vi "Keseluruhan Sistem.vi"() -> ()   [LabVIEW 2011]
doc: "The Basic Serial Read and Write example performs a Serial Port Read, a Serial Port Write, or a combination of these actions. The user selects the actions (read or write) on the front panel. If both are selected, the VI will write the data first, read data, and then close the VISA session that is opened to the port. This VI will wait until the specified number of bytes is received at the port. Only the number of bytes specified will be read.\n\nINSTRUCTIONS:\n1) Select the serial resource and configuration parameters (baud rate, data bits, parity, stop bits, flow control).\n2) Select the operations to be performed. \n3) Connect the serial port to your device. If no device is available, perform a loopback test by doing one of the following. Short pins 2 and 3 on a RS-232 cable or short pin 4 to pin 8 and pin 5 to pin 9 on a RS-485/422 cable. \n4) Run the VI to see the data read. (The \"read string\" will match the \"string to write\" if a loopback test was performed.)\n\nNote: The parameters set for the serial port must match the parameters of the connected instrument or device. In this example, the bytes to read parameter specifies the number of bytes that the serial port reads. If there were more bytes at the port than the number specified in bytes to read, those bytes would not be read. Also, if you specify to read more bytes than the number of bytes actually read, you might receive a timeout error message.\n\nOn the block diagram, the Configure Serial Port VI sets the configuration parameters. The front panel displays the controls used to configure the basic parameters, such as baud rate, data bits, and parity. Constants configure the other parameters the user probably does not need set. After the VISA Configure Serial Port VI opens the VISA session and configures the port, the VI passes the VISA resource name to other VIs that perform operations on that VISA resource. The VISA Write function sends a command to the serial device and the VISA Read function returns data based on the command. The VISA Close function then closes the reference to the serial device. It is important to close the reference; otherwise communication through with that port through protocols other than VISA might not be possible."
uses:
  <vilib>/Simulation/Scripting/Companion Diagram/SimConfigNode/SimParams.ctl
  <vilib>/Simulation/Scripting/Companion Diagram/SimConfigNode/_simSolvers.ctl
  <vilib>/Simulation/Implementation/Shared/SIMSCR Execution Mode.ctl
  <vilib>/Simulation/Param Hierarchy/Typedefs/SIMPH Param Control Actions.ctl
  <vilib>/Simulation/Implementation/Shared/NILVSim_FinalizeModel.vi
  <vilib>/Simulation/Implementation/Shared/NILVSim_Manager.vi
  <vilib>/Simulation/Implementation/Shared/NILVSim_ParamChanged.vi
  <vilib>/imath/engines/lvmath2/RunTimeEngine/ErrorHandling/NIMS_Finalize Error.vi
  <vilib>/imath/engines/lvmath2/RunTimeEngine/BuiltInFunctions/deg_to_rad/NIMS_deg_to_rad.vi
  <instcachedir>/0/NIMS_deg_to_rad_4A81D684CE8D4DD79924F5AB74D756E1.lvgen/NIMS_deg_to_rad_4A81D684CE8D4DD79924F5AB74D756E1_001.vi
  <vilib>/imath/engines/lvmath2/RunTimeEngine/NodeEndStatement/NIMS_NodeEndStatement_Output.vi
  <instcachedir>/0/NIMS_NodeEndStatement_Output_53EC0D466D134D7ABD903AC30B43404B.lvgen/NIMS_NodeEndStatement_Output_53EC0D466D134D7ABD903AC30B43404B_001.vi
  <instcachedir>/0/NIMS_NodeEndStatement_Output_53EC0D466D134D7ABD903AC30B43404B.lvgen/NIMS_NodeEndStatement_Output_53EC0D466D134D7ABD903AC30B43404B_012.vi
  <instcachedir>/0/NIMS_NodeEndStatement_Output_53EC0D466D134D7ABD903AC30B43404B.lvgen/NIMS_NodeEndStatement_Output_53EC0D466D134D7ABD903AC30B43404B_010.vi
  <vilib>/imath/engines/lvmath2/RunTimeSupport/NIMS_Complex To Real.vi
  <instcachedir>/0/NIMS_Complex To Real_C6C689ECDA084B0290AC275552CC3682.lvgen/NIMS_Complex To Real_C6C689ECDA084B0290AC275552CC3682_001.vi
  <vilib>/imath/engines/lvmath2/RunTimeEngine/BuiltInFunctions/rad_to_deg/NIMS_rad_to_deg.vi
  <instcachedir>/0/NIMS_rad_to_deg_A39AFCDDC8C049FCADAAB7FC30B9F5AA.lvgen/NIMS_rad_to_deg_A39AFCDDC8C049FCADAAB7FC30B9F5AA_001.vi
  <vilib>/imathl/engines/lvmath/Functions/Error Handling/Create Error.vi
  <vilib>/imath/engines/lvmath2/RunTimeEngine/BuiltInFunctions/abs/NIMS_abs(signed).vi
  <instcachedir>/0/NIMS_abs(signed)_C4FCB8E6058B49B797C7C8D53CA5F6EC.lvgen/NIMS_abs(signed)_C4FCB8E6058B49B797C7C8D53CA5F6EC_002.vi
  <vilib>/imath/engines/lvmath2/RunTimeEngine/BuiltInFunctions/acos/NIMS_acos(C).vi
  <instcachedir>/0/NIMS_acos(C)_7CE2F6FACE8F41D2AB6320A13102A19C.lvgen/NIMS_acos(C)_7CE2F6FACE8F41D2AB6320A13102A19C_001.vi
  <vilib>/Instr/_visa.llb/VISA Configure Serial Port (Instr).vi
  <vilib>/imath/engines/lvmath2/RunTimeEngine/Managers/WorkSpace/UID Generator.vi
  <vilib>/imath/engines/lvmath2/RunTimeEngine/Managers/SymbolTable/Clear UID.vi
  <instcachedir>/0/NIMS_abs(signed)_C4FCB8E6058B49B797C7C8D53CA5F6EC.lvgen/NIMS_abs(signed)_C4FCB8E6058B49B797C7C8D53CA5F6EC_007.vi
  <instcachedir>/0/NIMS_Complex To Real_C6C689ECDA084B0290AC275552CC3682.lvgen/NIMS_Complex To Real_C6C689ECDA084B0290AC275552CC3682_003.vi
  <vilib>/imath/engines/lvmath2/RunTimeEngine/RunTimeType/NIMS_RunTimeType_From StrictType (excl LVString).vi
  <instcachedir>/0/NIMS_RunTimeType_From StrictType (excl LVString)_46AE8B54A11948F0BCCEB8091EE7AA4C.lvgen/NIMS_RunTimeType_From StrictType (excl LVString)_46AE8B54A11948F0BCCEB8091EE7AA4C_000.vi
  <vilib>/imath/engines/lvmath2/RunTimeEngine/LocalVariableDefStatement/MC_LocalVariableDefStatement_Display.vi
  <vilib>/Simulation/Implementation/Shared/SIM Unbundle Sim Info.vi
  <vilib>/Simulation/Implementation/Shared/NILVSim_GetModelError.vi
  <vilib>/Simulation/Implementation/Shared/SIM Bundle Sim Info.vi
  <vilib>/Simulation/Implementation/Shared/NILVSim_Initialize.vi
  <vilib>/Simulation/Implementation/XNodeFramework/SimXNode/SimX.xnode
  <vilib>/Simulation/Model Libraries/PID/SIM PID (Academic).vi
  <vilib>/Simulation/Model Libraries/PID/SIM PID.vi
  <vilib>/Simulation/Scripting/Companion Diagram/SimConfigNode/SimDog.xnode
  <vilib>/vision/NI_Vision_Development_Module.lvlib
  <vilib>/Simulation/Implementation/Shared/NI_SIM_Implementation.lvlib
  <vilib>/imath/engines/lvmath2/RunTimeEngine/Managers/SymbolTable/NIMS_WorkSpace.lvlib
panel:
  in  "Color Plane":i32(ring)=1 items=["Red", "Green", "Blue", "Hue", "Saturation", "Luminance", "Value", "Intensity"]
  out "bytes read":u32
  out "read string":string
  out "error vision 2":errorcluster
  in  "STOP":bool caption="Stop (F)"
  out "error vision":errorcluster
  in  "OFFSET":dbl
  out "error out":errorcluster
  in  "error in":errorcluster
  in  "Tab Control":T1(tab)
  in  "Tab Control 2":T2(tab)
  in  "Tab Control 3":enum32{"Pengolahan Citra", "Kinematika"}(tab)
  in  "Settings":T3={"Objects"=1, "Threshold"=128, "Reject Border"=FALSE, "Fill Holes"=FALSE, "Min Object Size"=FALSE, "Min Size"=100, "Max Object Size"=FALSE, "Max Size"=10000, "Show Search Area"=FALSE, "Show Center"=TRUE, "Show Bounding Box"=TRUE} {"Objects" items=["Bright Objects", "Dark Objects"]; "Threshold" min=1 max=999999999 step=1; "Max Size" min=1 max=999999999 step=1; "Min Size" min=1 max=999999999 step=1}
  in  "Alamat Berkas":path=path "E:/D4 - TUGAS AKHIR/Programs/Praktikum/polman.png"
  out "Citra \nHitam/Putih":T4(plugin-control)
  out "Citra Asli":T4(plugin-control)
  out "Hasil\nSegmentasi":T4(plugin-control)
  out "Hasil \nKlasifikasi":T4(plugin-control)
  in  "BERKAS / KAMERA":bool
  out "Number of Objects":i32
  in  "Range":cluster{"Lower value":sgl, "Upper value":sgl}={"Lower value"=128.0, "Upper value"=255.0} {"Upper value" format="%.2f"; "Lower value" format="%.2f"}
  out "Objects":T5(array[cluster]) {"Aspect Ratio" format="%.2f"; "Orientation" format="%.2f"; "Area" format="%.2f"; "Object Center"."Y" format="%.2f"; "Object Center"."X" format="%.2f"}
  in  "Replace Value":sgl=255.0 format="%.2f"
  in  "Dimensi Lengan Robot":cluster{"l1":sgl, "l2":sgl, "l3":sgl, "l4":sgl}={"l1"=75.0, "l2"=95.0, "l3"=95.0, "l4"=107.0} caption="Arm Dimensiions 2"
  out "SIDE VIEW ROBOT":cluster{"Y":dbl[], "Y":dbl[]}[](graph)
  out "TOP VIEW ROBOT":cluster{"Y":dbl[], "Y":dbl[]}[](graph)
  in  "Kinematik Maju / Balik":enum32{"Kinematika Maju", "Kinematika Balik"}(tab)
  out "Koordinat Akhir (KM)":cluster{"X":dbl, "Y":dbl, "Z":dbl}
  in  "BASE":dbl(knob) scale=-90.0..90.0
  in  "SHOULDER":dbl(knob)=30.0 scale=0.0..135.0
  in  "ELBOW":dbl(knob)=150.0 scale=90.0..270.0
  in  "WRIST":dbl(knob)=150.0 scale=90.0..270.0
  in  "ELBOW CONFIG":bool
  in  "Koordinat Z":dbl(slide)=75.0 scale=0.0..300.0
  in  "Koordinat Y":dbl(slide) scale=-135.0..135.0
  in  "Koordinat X":dbl(slide)=297.0 scale=0.0..300.0
  out "Sudut Persendian (KB)":cluster{"q1":dbl, "q2":dbl, "q3":dbl, "q4":dbl}
  in  "theta":dbl(knob) scale=0.0..90.0
  in  "INTEGRATE":bool
  in  "PWM\nGRIPPER":i32
  in  "SETPOINT\nGAYA":dbl=35.0
  in  "FREEZE":bool caption="Stop (F)"
  in  "INITIAL":bool caption="Stop (F)"
  out "SIDE VIEW":cluster{"Y":dbl[], "Y":dbl[]}[](graph)
  in  "Drawing Mode":u32(ring) items=["Frame", "Fill", "Highlight"]
  out "Image":T4(plugin-control)
  in  "Color":u32(colorbox)=16711680
  out "Waveform Chart":dynamicdata(graph)
  in  "Arm Dimensiions":cluster{"l1":sgl, "l2":sgl, "l3":sgl, "l4":sgl}={"l1"=75.0, "l2"=95.0, "l3"=95.0, "l4"=107.0} caption="Arm Dimensiions 2"
  out "PWM Values":T6
  out "Joint Angles":cluster{"q1":dbl, "q2":dbl, "q3":dbl, "q4":dbl}
  in  "START":bool
  in  "buffer":string
  out "TOP VIEW":cluster{"Y":dbl[], "Y":dbl[]}[](graph)
  out "Z ROBOT":sgl
  out "Y ROBOT":sgl
  out "X ROBOT":sgl
  out "Z CAMERA":sgl
  out "X CAMERA":sgl
  out "Y CAMERA":sgl
  in  "WAIT TIME":u32=750
  in  "VISA NAME":refnum<visa-resource-name>="COM24"
  out "SHADOW":sgl
  in  "INDICATOR":bool
  in  "FORCE \nCONTROL":bool
  in  "SETPOINT\nPOSISI":i32=1250
  out "OUTPUT":dbl
  in  "Kp":dbl=0.7
  in  "Ti":dbl=1.55
  in  "Td":dbl
  in  "ERROR":dbl
  out "INPUT":u8
  # "Rancang Bangun Sistem Kendali Pergerakan Berbasis Pengolahan Citra \ndan Kendali Gaya Pencekaman Pada Model Robot Berlengan\nNur Jamiludin R. , Dr. Noval Lilansa, Dipl. Ing., MT. , Afaf Fadhil Rifa'i, ST. MT.\nJurusan Teknik Mesin dan Manufaktur Konsentrasi Teknik Elektromekanik.\nPoliteknik Manufaktur Negeri Bandung\nJl. Kanayakan No. 21, Bandung 40135\nINDONESIA\nEmail : nur_jamiludin@elmecs-indonesia.com"
  # "Deskripsi\n\nSebuah robot berlengan mampu melakukan pekerjaan pemindahan obyek. Kebanyakan robot memiliki waktu operasi yang tidak efisien karena membutuhkan proses masukan koordinat tujuan oleh operator. Selain permasalahan tersebut masalah robot berlengan terbesar ialah bahwa saat robot melakukan tugas pemindahan obyek, robot tersebut berpotensi merusak obyek yang dipindahkan. Dibutuhkan sistem kendali pergerakan robot yang memiliki kemampuan pendeteksian obyek berbasis pengolahan citra, sehingga robot mampu menentukan koordinat tujuan secara otomatis. \n\nProgram ini merupakan program pengendali model robot berlengan lynxmotion L5AC yang terintegrasi pada sebuah kamera dengan resolusi 3.0 Megapixel dan perangkat keras SSC (Serial Servo Controller). Program kendali robot berlengan ini bertujuan mengendalikan sistem agar dapat mendeteksi obyek berbentuk bola secara otomatis, serta dapat memindahkan obyek tersebut tanpa menimbulkan cacat bentuk pada objek."
  # "Citra asli hasil \ntangkapan kamera"
  # "Berkaitan dengan persiapan pengolahan citra. \nIdentifikasi spesifikasi resolusi kamera\nPenentuan peletakkan titik pusat lensa kamera\nPenentuan ukuran hasil citra (image) yang diambil"
  # "Prepocessing"
  # "hasil segmentasi"
  # "Segmentasi menggunakan metode tresholding.\nProses tresholding mengubah citra dengan format gray-scale menjadi citra biner untuk memisahkan obyek pada citra dengan latar belakangnya."
  # "Segmentasi"
  # "Koordinat obyek hasil estimasi posisi merupakan koordinat dengan titik pusat area kerja sebagai referensi\nPindahkan referensinya menjadi titik pusat robot sebagai referensi"
  # "hasil klasifikasi"
  # "Ekstraksi ciri mencari obyek dengan karakteristik tertentu dari data citra yang diperoleh. \nKlasifikasi menentukan obyek dari informasi citra yang diolah dengan perhitungan matematis berdasarkan karakter fisik obyek."
  # "Ekstraksi Ciri\ndan Klasifikasi"
  # "Estimasi posisi  mendapatkan vektor posisi pusat massa obyek  terhadap pusat kerangka koordinat area kerja. \nKemudian dilakukan translasi pusat kerangka koordinat area kerja ke pusat kerangka koordinat base robot,"
  # "Estimasi Posisi"
  # "hasil estimasi posisi"
  # "Transformasi Homogen"
  # "tentukan kerangka koordinat tiap joint"
  # "konstruksi model robot"
  # "tentukan panjang link dan link offset"
  # "Parameter D-H\n(Denavit-Hattenberg)"
  # "tentukan link twist , joint angle merupakan variable"
  # "pemodelan stick diagram"
  # "Algoritma Perhitungan Matrix"
  # "Analisa Geometri"
  # "Pengendalian gaya yang digunakan pada sistem pada dasarnya merupakan pengendalian posisi bukaan gripper\nPosisi bukaan gripper merupakan fungsi dari gaya yang diakuisisi oleh sensor dikali dengan koefisien peredam (damper). pada sistem kendali dalam tugas akhir ini, koefisien peredam yang dimaksud merupakan karakteristik mekanik dari model lengan robot yang digunakan.\nPengendalian posisi dipilih mengingat penggerak gripper merupakan motor servo yang bergerak berdasarkan setpoint posisi."
  # "Percobaan kinematika maju ini didasarkan pada konfigurasi robot berlengan yang terintegrasi dengan sistem. \nRobot yang digunakan merupakan robot revolute yang memiliki 4 DOF ditambah satu gripper.\nRentang sudut yang diperbolehkan juga berdasarkan karakteristik penggerak robot\n\nParameter D-H  robot dapat dilihat pada tabel disamping."
  # "Percobaan kinematika balik ini merupakan perhitungan balik dari \npercobaan kinematika maju pada tab sebelumnya.\nsolusi kinematika balik yang beragam ditampilkan pada simulasi\ndengan memilih konfigurasi elbow up atau elbow down \nnamun robot berlengan yang terintegrasi dengan sistem hanya \nmenggunakan konfigurasi elbow up"
  # "mm"
  # "mm"
  # "mm"
  # "mm"
  # "mm"
  # "mm"
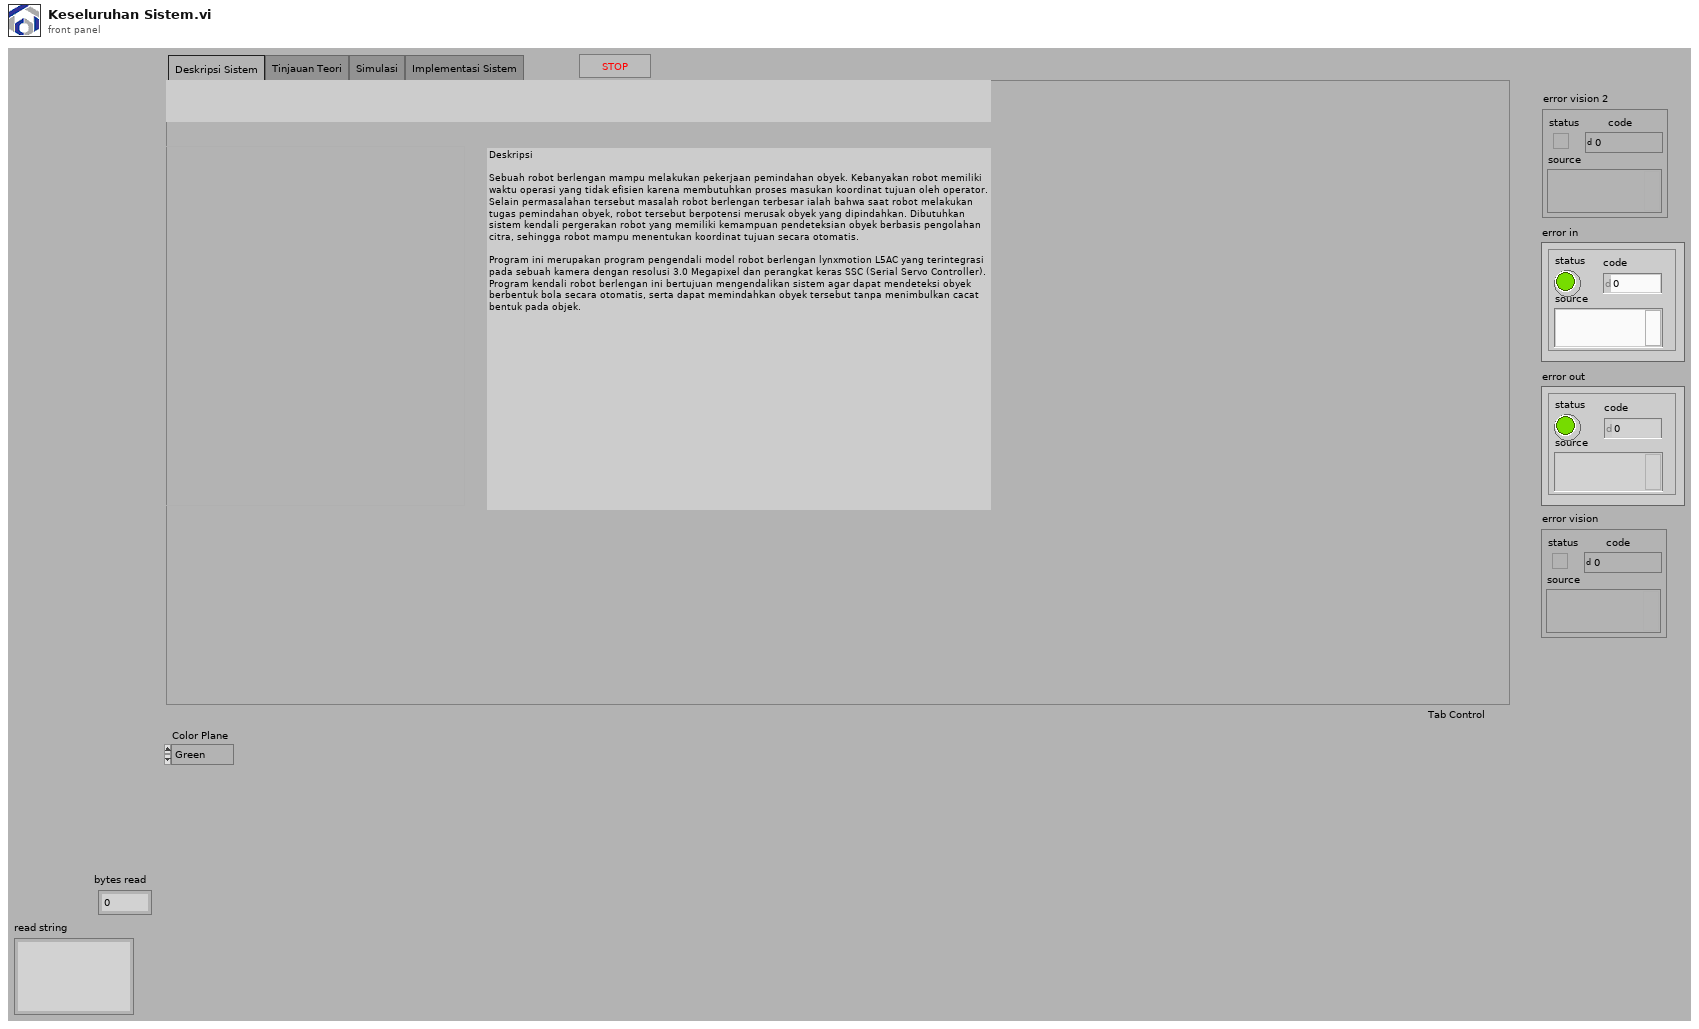
[diagram p1: front panel]
types:
  T1 = enum32{"Deskripsi Sistem", "Tinjauan Teori", "Simulasi", "Implementasi Sistem"}
  T2 = enum32{"Pengolahan Citra", "Kinematika Maju", "Kinematika Balik", "Pengendalian Gaya"}
  T3 = cluster{"Objects":u16, "Threshold":i32, "Reject Border":bool, "Fill Holes":bool, "Min Object Size":bool, "Min Size":i32, "Max Object Size":bool, "Max Size":i32, "Show Search Area":bool, "Show Center":bool, "Show Bounding Box":bool}
  T4 = typedef "IMAQ Image.ctl" = refnum<image>
  T5 = cluster{"Object Center":cluster{"X":sgl, "Y":sgl}, "Bounding Box":cluster{"X Left":i32, "Y Top":i32, "X Right":i32, "Y Bottom":i32}, "Area":sgl, "Orientation":sgl, "Aspect Ratio":sgl, "Nb Holes":i32}[]
  T6 = cluster{"PWM1":u32, "PWM2":u32, "PWM3":u32, "PWM4":u32}
  T7 = typedef "Image Type" = u32
  T8 = typedef "SIMPH Param Control Actions.ctl" = enum16{"get params", "set params"}
  T9 = typedef "SimParams.ctl" = cluster{"Initial Time (s)":dbl, "Final Time (s)":dbl, "Step Size (s)":dbl, "ODE Solver":T10, "Minimum Step Size (s)":dbl, "Maximum Step Size (s)":dbl, "Relative Tolerance":dbl, "Absolute Tolerance":dbl, "Software Timing":bool, "Initial Step Size (s)":dbl, "Automatic Fixed Step Size?":bool, "Automatic Discrete Step Size?":bool, "Discrete Step Size (s)":dbl, "Calculate using Time Step":bool, "Solver Wired?":bool, "Prev.Frm.Expected End":u64, "Prev.Frm.Actual End":u64, "Prev.Frm.Finished Late?":bool, "Prev.Iter.Expected End":u64, "Prev.Iter.Actual End":u64, "Prev.Iter.Finished Late?":bool, "Expected Iteration Start":u64, "Actual Iteration Start":u64, "Expected Frame Start":u64, "Actual Frame Start":u64, "Source Name":string, "Name":string, "Period":i64, "Deadline":i64, "Offset":i64, "Start":i64, "Priority":i32, "Timeout":i32, "Processor":i32, "Mode":enum32{"No Change", "Process missed periods, maintain original phase", "Discard missed periods, maintain original phase", "Process missed periods, ignore original phase", "Discard missed periods, ignore original phase"}, "Wakeup reason":enum32{"Normal", "Aborted", "Asynchronous wakeup", "Timing source error", "Timed loop error", "Timeout"}, "Error":errorcluster, "Source Type":string, "Secondary Source Type":string, "Global End Time":u64, "Global Start Time":u64, "Full Solver Reset":bool, "Execution Mode":T11, "Nan/Inf Check":bool, "Custom Solver Library":string, "Solver Is Variable":bool, "custom solver name":string}
  T10 = typedef "_simSolvers.ctl" = enum16{"Runge-Kutta 1 (Euler)", "Runge-Kutta 2", "Runge-Kutta 3", "Runge-Kutta 4", "Runge-Kutta 23 (variable)", "Runge-Kutta 45 (variable)", "BDF (variable)", "Adams-Moulton (variable)", "Rosenbrock (variable)", "Discrete States Only", "Linearizer", "State Query", "Trim Eval", "Custom Solver"}
  T11 = typedef "SIMSCR Execution Mode.ctl" = u16
  T12 = cluster{"PW1":u32, "PW2":u32, "PW3":u32, "PW4":u32}
  T13 = cluster{"Theta1":dbl, "Theta2":dbl, "Theta3":dbl, "Theta4":dbl}
  T14 = cluster{"Theta0":dbl, "Theta1":dbl, "Theta2":dbl}
  T15 = cluster{"Theta0":dbl, "Theta1":dbl, "Theta2":dbl, "Theta3":dbl}
  T16 = cluster{"Edge Coordinates (horizontal)[0]":cluster{"X":sgl, "Y":sgl}, "Edge Coordinates (horizontal)[1]":cluster{"X":sgl, "Y":sgl}, "Edge Coordinates (horizontal)[2]":cluster{"X":sgl, "Y":sgl}, "Edge Coordinates (horizontal)[3]":cluster{"X":sgl, "Y":sgl}, "Edge Coordinates (horizontal)[4]":cluster{"X":sgl, "Y":sgl}, "Edge Coordinates (horizontal)[5]":cluster{"X":sgl, "Y":sgl}, "Edge Coordinates (horizontal)[6]":cluster{"X":sgl, "Y":sgl}, "Edge Coordinates (horizontal)[7]":cluster{"X":sgl, "Y":sgl}}
  T17 = cluster{"Edge Coordinates (vertical)[0]":cluster{"X":sgl, "Y":sgl}, "Edge Coordinates (vertical)[1]":cluster{"X":sgl, "Y":sgl}, "Edge Coordinates (vertical)[2]":cluster{"X":sgl, "Y":sgl}, "Edge Coordinates (vertical)[3]":cluster{"X":sgl, "Y":sgl}, "Edge Coordinates (vertical)[4]":cluster{"X":sgl, "Y":sgl}, "Edge Coordinates (vertical)[5]":cluster{"X":sgl, "Y":sgl}, "Edge Coordinates (vertical)[6]":cluster{"X":sgl, "Y":sgl}, "Edge Coordinates (vertical)[7]":cluster{"X":sgl, "Y":sgl}}
  T18 = cluster{"unsigned byte array[0]":u8, "unsigned byte array[1]":u8, "unsigned byte array[2]":u8, "unsigned byte array[3]":u8, "unsigned byte array[4]":u8, "unsigned byte array[5]":u8, "unsigned byte array[6]":u8, "unsigned byte array[7]":u8, "unsigned byte array[8]":u8, "unsigned byte array[9]":u8, "unsigned byte array[10]":u8, "unsigned byte array[11]":u8, "unsigned byte array[12]":u8, "unsigned byte array[13]":u8, "unsigned byte array[14]":u8, "unsigned byte array[15]":u8, "unsigned byte array[16]":u8, "unsigned byte array[17]":u8}
  T19 = cluster{"[0]":sgl, "[1]":sgl, "[2]":sgl, "[3]":sgl}
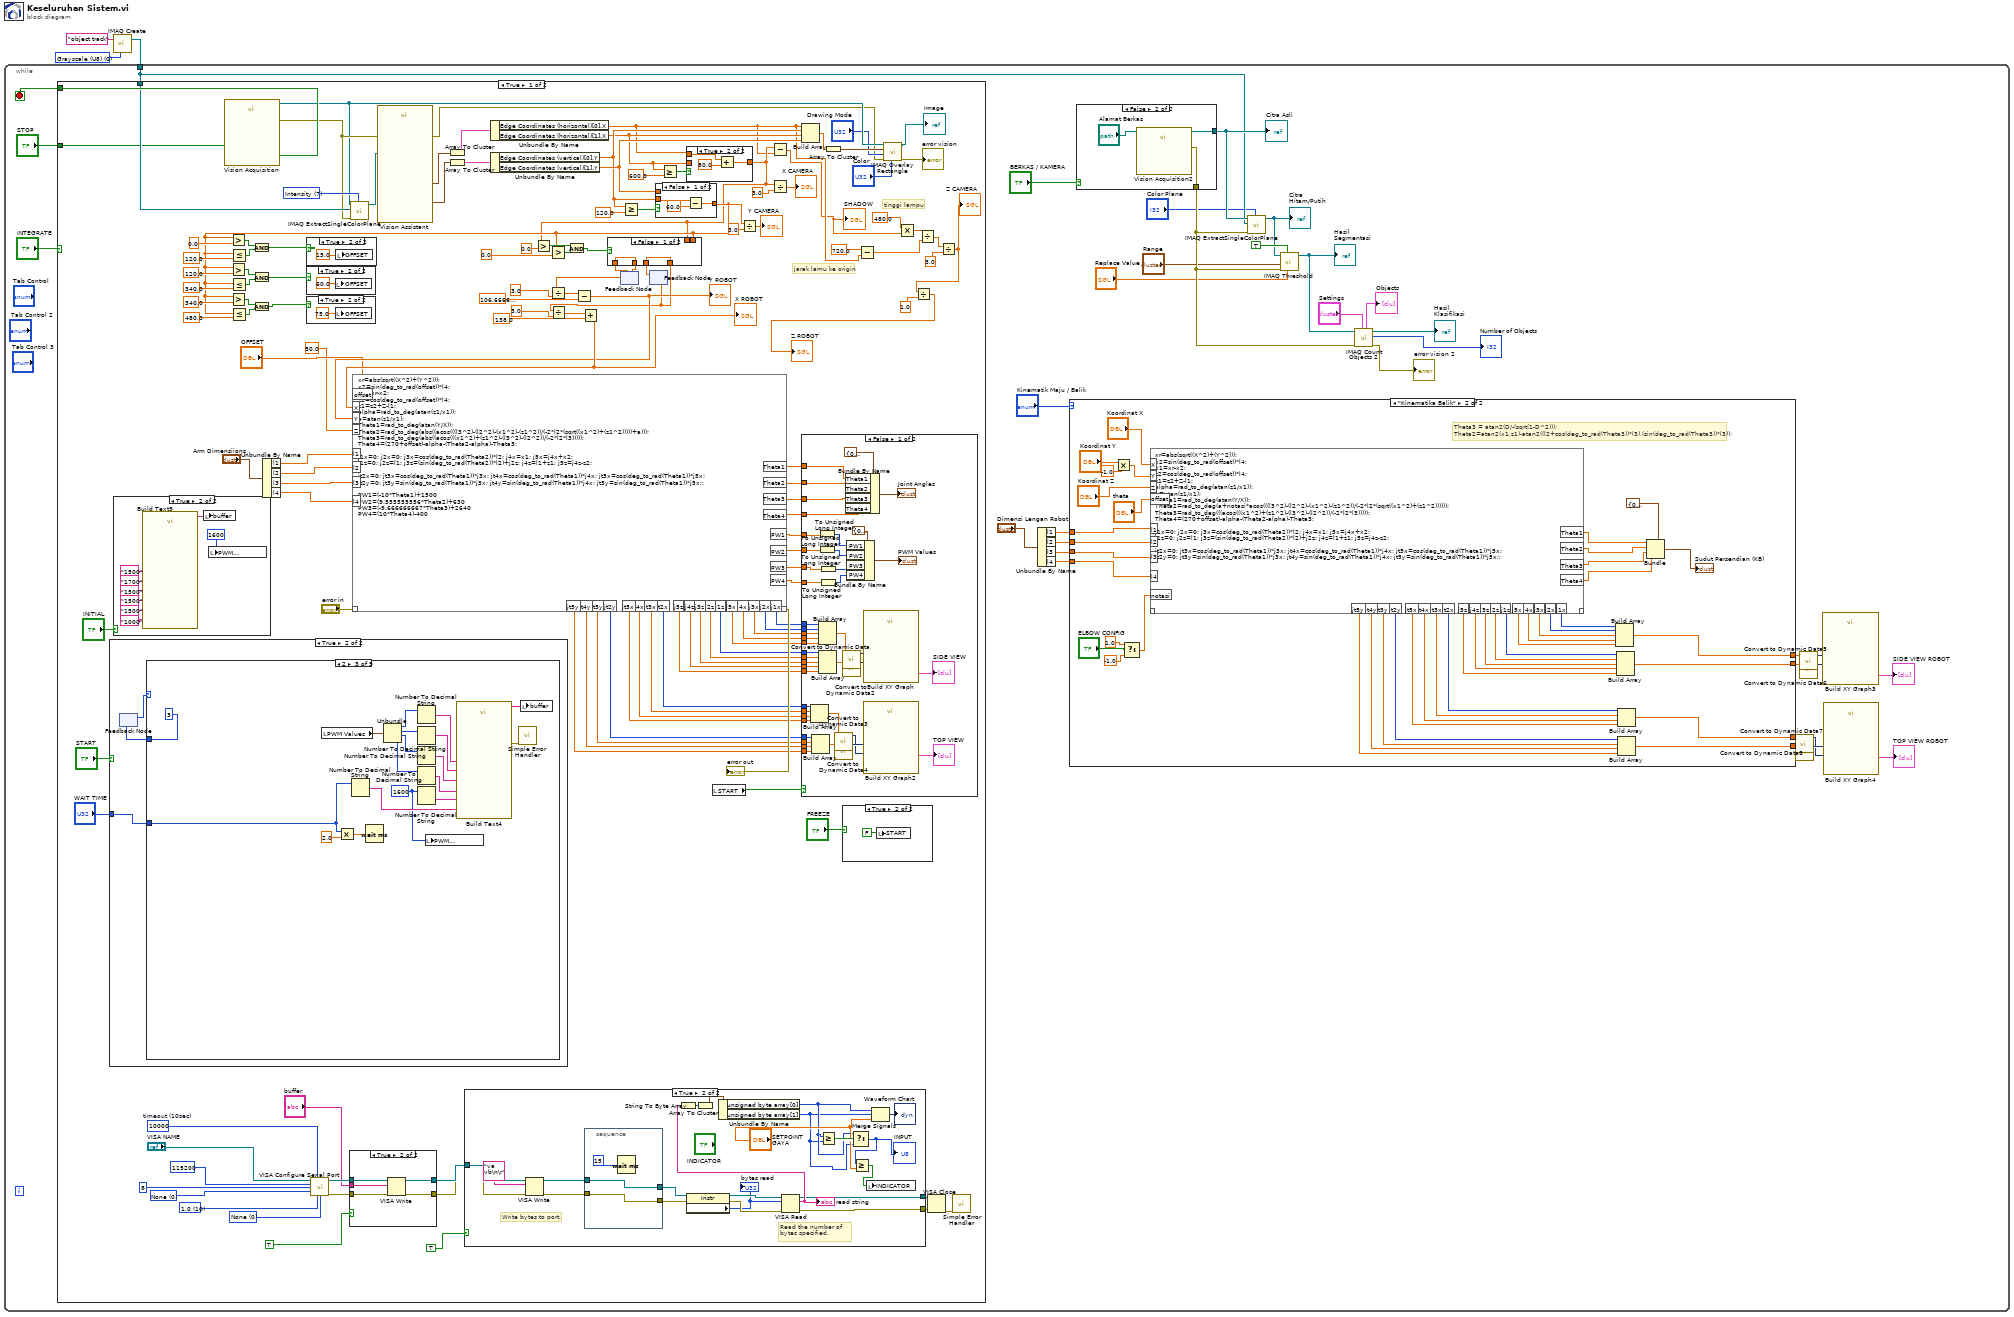
[diagram p0: block diagram]
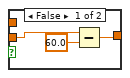
[diagram p4: hidden frame]
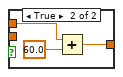
[diagram p6: hidden frame]
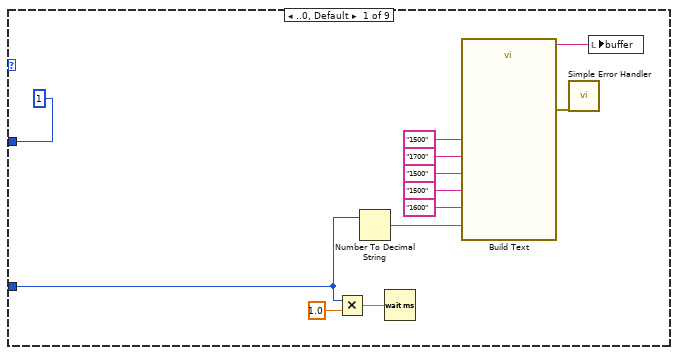
[diagram p11: hidden frame]
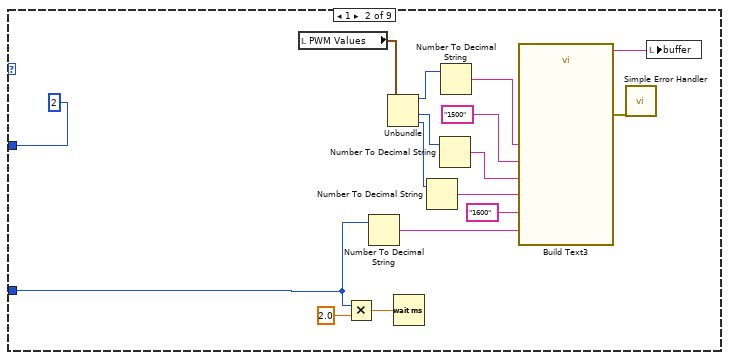
[diagram p12: hidden frame]
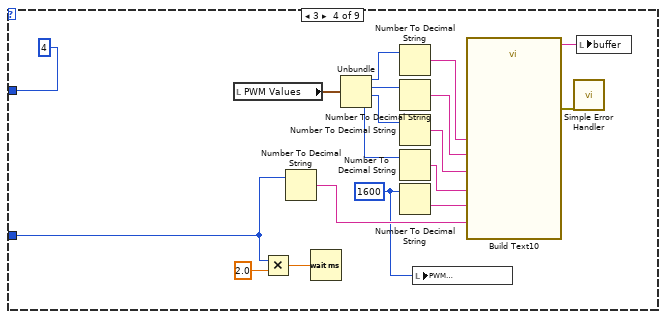
[diagram p13: hidden frame]
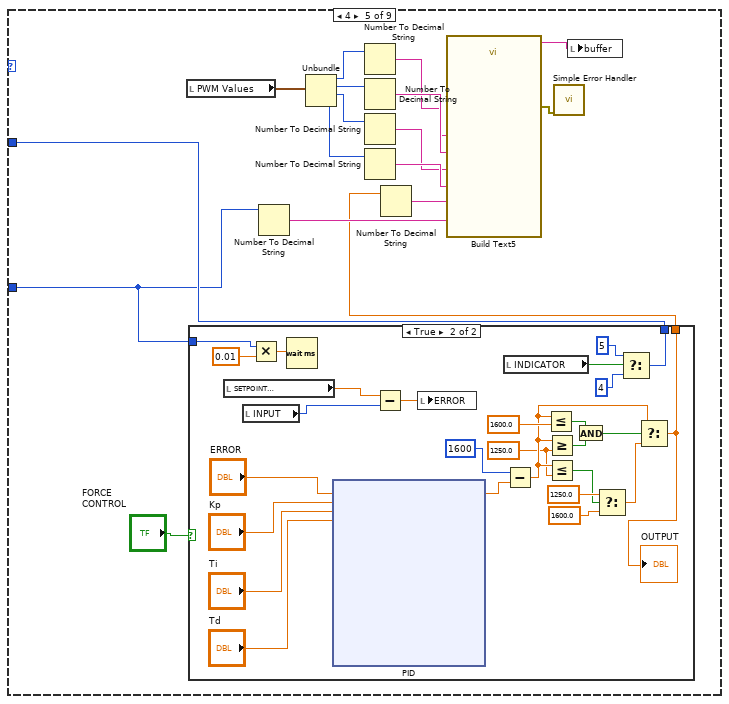
[diagram p14: hidden frame]
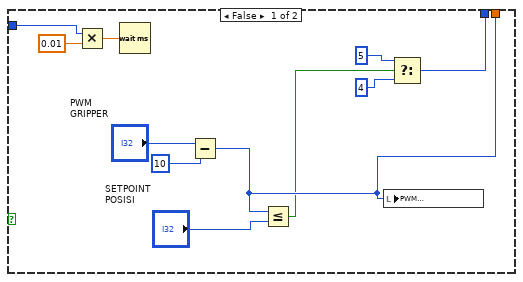
[diagram p15: hidden frame]
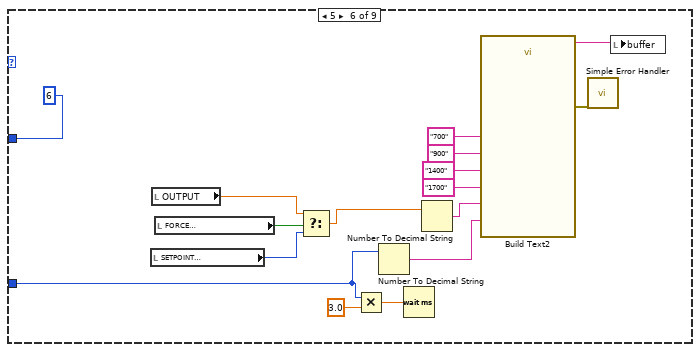
[diagram p16: hidden frame]
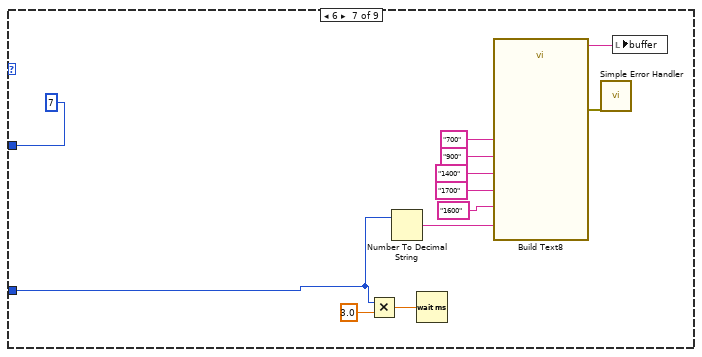
[diagram p17: hidden frame]
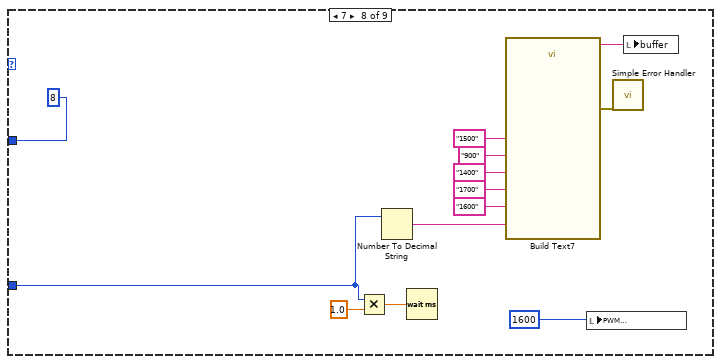
[diagram p18: hidden frame]
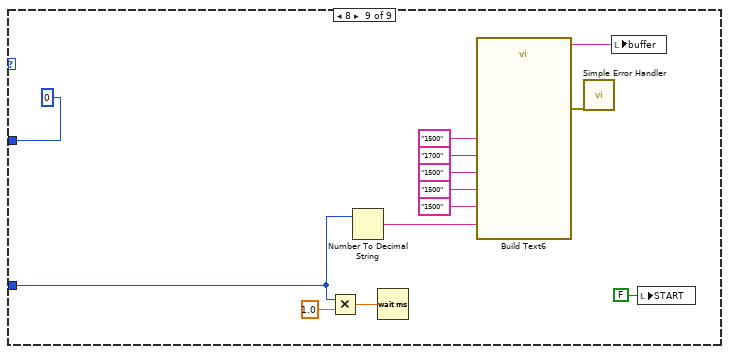
[diagram p19: hidden frame]
diagram:
  w2 = T7 0 items=["Grayscale (U8)", "Grayscale (I16)", "Grayscale (SGL)", "Complex (CSG)", "RGB (U32)", "HSL (U32)", "RGB (U64)", "Grayscale (U16)"] ("Image Type")
  n1 = call "IMAQ Create"("Image Name"="object track", "Image Type"=w2) -> ("New Image"=w1:T4)  [unwired: 3 in, 1 out]
  n2 = while {
    tunnel: w1 -> [w10]
    stop <- w37 stop-if-true
    n3 = case shown="True" "INTEGRATE" {
      tunnel: [w168 w1024] -> w37
      tunnel: w10 -> [w167 _]
      tunnel: "STOP" -> [w83 w1024]
      frame True {
        w141 = u16 0 items=["None"=0, "XON/XOFF"=1, "RTS/CTS"=2, "DTR/DSR"=4] ("flow control")
        w142 = u16 10 items=["1.0"=10, "1.5"=15, "2.0"=20] ("stop bits")
        w144 = u16 0 items=["None", "Odd", "Even", "Mark", "Space"] ("parity")
        w143 = u32 10000  # timeout (10sec)
        w166 = 7 items=["Red", "Green", "Blue", "Hue", "Saturation", "Luminance", "Value", "Intensity"] ("Color Plane")
        # "tinggi lampu"
        # "jarak lamu ke origin"
        # "Enter constants for your servo calibrations here"
        n4 = case shown="True" "START" {
          tunnel: "WAIT TIME" -> [_ w222]
          frame False {
          }
          frame True {
            n5 = feedback #1() -> (w220:i32)  [unwired: 1 in]
            n6 = case shown="2" w220 {
              tunnel: w222 -> [w224 w245 w254 w272 w296 w477 w489 w500 w512]
              tunnel: [1 ("Numeric") 2 ("Numeric") 3 ("Numeric") 4 ("Numeric") w297 6 ("Numeric") 7 ("Numeric") 8 ("Numeric") 0 ("Numeric")] -> w221
              frame ..0, Default {
                n7 = Multiply(x=w224, y=1.0) -> (x*y=w226:dbl)
                n8 = Number To Decimal String(number=w224) -> (decimal integer string=w225:string)  [unwired: 1 in]
                n9 = Wait (ms)(milliseconds to wait=w226) -> ()  [unwired: 1 out]
                n10 = call "Build Text"("pwm3"="1500", "time"=w225, "pwm0"="1500", "pwm1"="1700", "pwm2"="1500", "pwm4"="1600") -> ("Result"=w228:string, "error out"=w234:errorcluster)  [unwired: 8 in]
                n11 = call <vilib>:"Simple Error Handler.vi"("error in (no error)"=w234) -> ()  [unwired: 4 in, 5 out]
                n12 = local write "buffer"(w228) -> ()
              }
              frame 1 {
                n13 = local read "PWM Values"() -> (w241:T6)
                n14 = Multiply(x=w245, y=2.0) -> (x*y=w246:dbl)
                n15 = Number To Decimal String(number=w245) -> (decimal integer string=w244:string)  [unwired: 1 in]
                n16 = Unbundle(w241) -> ("PWM1"=w243:u32, "PWM3"=w238:u32, "PWM4"=w239:u32)  [unwired: 1 out]
                n17 = Wait (ms)(milliseconds to wait=w246) -> ()  [unwired: 1 out]
                n18 = Number To Decimal String(number=w239) -> (decimal integer string=w240:string)  [unwired: 1 in]
                n19 = Number To Decimal String(number=w238) -> (decimal integer string=w237:string)  [unwired: 1 in]
                n20 = Number To Decimal String(number=w243) -> (decimal integer string=w242:string)  [unwired: 1 in]
                n21 = call "Build Text3"("pwm3"=w240, "time"=w244, "pwm0"=w242, "pwm1"="1500" ("pwm3"), "pwm2"=w237, "pwm4"="1600") -> ("Result"=w248:string, "error out"=w250:errorcluster)  [unwired: 8 in]
                n22 = call <vilib>:"Simple Error Handler.vi"("error in (no error)"=w250) -> ()  [unwired: 4 in, 5 out]
                n23 = local write "buffer"(w248) -> ()
              }
              frame 2 {
                w252 = 1600 ("number")
                n24 = local read "PWM Values"() -> (w260:T6)
                n25 = Multiply(x=w254, y=2.0) -> (x*y=w255:dbl)
                n26 = Number To Decimal String(number=w254) -> (decimal integer string=w253:string)  [unwired: 1 in]
                n27 = Wait (ms)(milliseconds to wait=w255) -> ()  [unwired: 1 out]
                n28 = Unbundle(w260) -> ("PWM1"=w265:u32, "PWM2"=w266:u32, "PWM3"=w267:u32, "PWM4"=w268:u32)
                n29 = Number To Decimal String(number=w265) -> (decimal integer string=w259:string)  [unwired: 1 in]
                n30 = Number To Decimal String(number=w266) -> (decimal integer string=w261:string)  [unwired: 1 in]
                n31 = Number To Decimal String(number=w267) -> (decimal integer string=w262:string)  [unwired: 1 in]
                n32 = Number To Decimal String(number=w268) -> (decimal integer string=w263:string)  [unwired: 1 in]
                n33 = Number To Decimal String(number=w252) -> (decimal integer string=w264:string)  [unwired: 1 in]
                n34 = local write "PWM\nGRIPPER"(w252) -> ()
                n35 = call "Build Text4"("pwm3"=w263, "time"=w253, "pwm0"=w259, "pwm1"=w261, "pwm2"=w262, "pwm4"=w264) -> ("Result"=w258:string, "error out"=w257:errorcluster)  [unwired: 8 in]
                n36 = call <vilib>:"Simple Error Handler.vi"("error in (no error)"=w257) -> ()  [unwired: 4 in, 5 out]
                n37 = local write "buffer"(w258) -> ()
              }
              frame 3 {
                w270 = 1600 ("number")
                n38 = local read "PWM Values"() -> (w278:T6)
                n39 = Multiply(x=w272, y=2.0) -> (x*y=w273:dbl)
                n40 = Number To Decimal String(number=w272) -> (decimal integer string=w271:string)  [unwired: 1 in]
                n41 = Wait (ms)(milliseconds to wait=w273) -> ()  [unwired: 1 out]
                n42 = Unbundle(w278) -> ("PWM1"=w283:u32, "PWM2"=w284:u32, "PWM3"=w285:u32, "PWM4"=w286:u32)
                n43 = Number To Decimal String(number=w283) -> (decimal integer string=w277:string)  [unwired: 1 in]
                n44 = Number To Decimal String(number=w284) -> (decimal integer string=w279:string)  [unwired: 1 in]
                n45 = Number To Decimal String(number=w285) -> (decimal integer string=w280:string)  [unwired: 1 in]
                n46 = Number To Decimal String(number=w286) -> (decimal integer string=w281:string)  [unwired: 1 in]
                n47 = Number To Decimal String(number=w270) -> (decimal integer string=w282:string)  [unwired: 1 in]
                n48 = local write "PWM\nGRIPPER"(w270) -> ()
                n49 = call "Build Text10"("pwm3"=w281, "time"=w271, "pwm0"=w277, "pwm1"=w279, "pwm2"=w280, "pwm4"=w282) -> ("Result"=w276:string, "error out"=w275:errorcluster)  [unwired: 8 in]
                n50 = call <vilib>:"Simple Error Handler.vi"("error in (no error)"=w275) -> ()  [unwired: 4 in, 5 out]
                n51 = local write "buffer"(w276) -> ()
              }
              frame 4 {
                n52 = local read "PWM Values"() -> (w287:T6)
                n53 = case shown="True" "FORCE \nCONTROL" {
                  tunnel: [w308 w336] -> w297
                  tunnel: [w312 w327] -> w298
                  tunnel: w296 -> [w304 w322]
                  frame False {
                    n54 = Multiply(x=w304, y=0.01) -> (x*y=w305:dbl)
                    n55 = Wait (ms)(milliseconds to wait=w305) -> ()  [unwired: 1 out]
                    n56 = Subtract(x="PWM\nGRIPPER", y=10) -> (x-y=w312:i32)
                    n57 = Less Or Equal?(x=w312, y="SETPOINT\nPOSISI") -> (x <= y?=w310:bool)
                    n58 = local write "PWM\nGRIPPER"(w312) -> ()
                    n59 = Select(t=5, s=w310, f=4 ("t")) -> (s? t:f=w308:i32)
                  }
                  frame True {
                    w317 = 1250.0 ("x")
                    n60 = local read "SETPOINT\nGAYA"() -> (w326:dbl)
                    n61 = local read "INPUT"() -> (w315:u8)
                    n62 = Multiply(x=w322, y=0.01) -> (x*y=w323:dbl)
                    n63 = Wait (ms)(milliseconds to wait=w323) -> ()  [unwired: 1 out]
                    n64 = xnode "PID"("Error"="ERROR", "Proportional Gain (Kc)"="Kp", "Integral time [s] (Ti)"="Ti", "Derivative time [s] (Td)"="Td") -> ("Output"=w334:dbl)  [unwired: 2 in, 11 out]
                    n65 = Subtract(x=w326, y=w315) -> (x-y=w316:dbl)
                    n66 = local write "ERROR"(w316) -> ()
                    n67 = local read "INDICATOR"() -> (w333:bool)
                    n68 = Subtract(x=1600, y=w334) -> (x-y=w318:dbl)
                    n69 = Less Or Equal?(x=w318, y=1600.0 ("x")) -> (x <= y?=w331:bool)
                    n70 = Greater Or Equal?(x=w318, y=w317) -> (x >= y?=w329:bool)
                    n71 = Less Or Equal?(x=w318, y=w317) -> (x <= y?=w319:bool)
                    n72 = And(x=w331, y=w329) -> (x .and. y?=w330:bool)
                    n73 = Select(t=1250.0 ("f"), s=w319, f=1600.0) -> (s? t:f=w328:dbl)
                    n74 = Select(t=5 ("Numeric"), s=w333, f=4 ("Numeric")) -> (s? t:f=w336:i32)
                    n75 = Select(t=w318, s=w330, f=w328) -> (s? t:f=w327:dbl)
                    "OUTPUT" <- w327
                  }
                }
                n76 = Number To Decimal String(number=w296) -> (decimal integer string=w302:string)  [unwired: 1 in]
                n77 = Unbundle(w287) -> ("PWM1"=w292:u32, "PWM2"=w293:u32, "PWM3"=w294:u32, "PWM4"=w295:u32)
                n78 = Number To Decimal String(number=w292) -> (decimal integer string=w288:string)  [unwired: 1 in]
                n79 = Number To Decimal String(number=w293) -> (decimal integer string=w289:string)  [unwired: 1 in]
                n80 = Number To Decimal String(number=w294) -> (decimal integer string=w290:string)  [unwired: 1 in]
                n81 = Number To Decimal String(number=w295) -> (decimal integer string=w291:string)  [unwired: 1 in]
                n82 = Number To Decimal String(number=w298) -> (decimal integer string=w300:string)  [unwired: 1 in]
                n83 = call "Build Text5"("pwm3"=w291, "time"=w302, "pwm0"=w288, "pwm1"=w289, "pwm2"=w290, "pwm4"=w300) -> ("Result"=w303:string, "error out"=w301:errorcluster)  [unwired: 8 in]
                n84 = call <vilib>:"Simple Error Handler.vi"("error in (no error)"=w301) -> ()  [unwired: 4 in, 5 out]
                n85 = local write "buffer"(w303) -> ()
              }
              frame 5 {
                n86 = local read "SETPOINT\nPOSISI"() -> (w472:i32)
                n87 = local read "OUTPUT"() -> (w473:dbl)
                n88 = local read "FORCE \nCONTROL"() -> (w474:bool)
                n89 = Select(t=w473, s=w474, f=w472) -> (s? t:f=w471:dbl)
                n90 = Multiply(x=w477, y=3.0) -> (x*y=w479:dbl)
                n91 = Number To Decimal String(number=w477) -> (decimal integer string=w478:string)  [unwired: 1 in]
                n92 = Wait (ms)(milliseconds to wait=w479) -> ()  [unwired: 1 out]
                n93 = Number To Decimal String(number=w471) -> (decimal integer string=w475:string)  [unwired: 1 in]
                n94 = call "Build Text2"("pwm3"="1700", "time"=w478, "pwm0"="700", "pwm1"="900", "pwm2"="1400", "pwm4"=w475) -> ("Result"=w476:string, "error out"=w485:errorcluster)  [unwired: 8 in]
                n95 = call <vilib>:"Simple Error Handler.vi"("error in (no error)"=w485) -> ()  [unwired: 4 in, 5 out]
                n96 = local write "buffer"(w476) -> ()
              }
              frame 6 {
                n97 = Multiply(x=w489, y=3.0) -> (x*y=w491:dbl)
                n98 = Number To Decimal String(number=w489) -> (decimal integer string=w490:string)  [unwired: 1 in]
                n99 = Wait (ms)(milliseconds to wait=w491) -> ()  [unwired: 1 out]
                n100 = call "Build Text8"("pwm3"="1700", "time"=w490, "pwm0"="700", "pwm1"="900", "pwm2"="1400", "pwm4"="1600") -> ("Result"=w487:string, "error out"=w497:errorcluster)  [unwired: 8 in]
                n101 = call <vilib>:"Simple Error Handler.vi"("error in (no error)"=w497) -> ()  [unwired: 4 in, 5 out]
                n102 = local write "buffer"(w487) -> ()
              }
              frame 7 {
                n103 = Multiply(x=w500, y=1.0) -> (x*y=w503:dbl)
                n104 = Number To Decimal String(number=w500) -> (decimal integer string=w502:string)  [unwired: 1 in]
                n105 = Wait (ms)(milliseconds to wait=w503) -> ()  [unwired: 1 out]
                n106 = call "Build Text7"("pwm3"="1700", "time"=w502, "pwm0"="1500", "pwm1"="900", "pwm2"="1400", "pwm4"="1600") -> ("Result"=w501:string, "error out"=w510:errorcluster)  [unwired: 8 in]
                n107 = local write "PWM\nGRIPPER"(1600 ("number")) -> ()
                n108 = call <vilib>:"Simple Error Handler.vi"("error in (no error)"=w510) -> ()  [unwired: 4 in, 5 out]
                n109 = local write "buffer"(w501) -> ()
              }
              frame 8 {
                n110 = Multiply(x=w512, y=1.0) -> (x*y=w514:dbl)
                n111 = Number To Decimal String(number=w512) -> (decimal integer string=w513:string)  [unwired: 1 in]
                n112 = Wait (ms)(milliseconds to wait=w514) -> ()  [unwired: 1 out]
                n113 = call "Build Text6"("pwm3"="1500", "time"=w513, "pwm0"="1500", "pwm1"="1700", "pwm2"="1500", "pwm4"="1500") -> ("Result"=w517:string, "error out"=w523:errorcluster)  [unwired: 8 in]
                n114 = call <vilib>:"Simple Error Handler.vi"("error in (no error)"=w523) -> ()  [unwired: 4 in, 5 out]
                n115 = local write "buffer"(w517) -> ()
                n116 = local write "START"(FALSE ("START")) -> ()
              }
            }
            n117 = feedback-in #1(w221) -> ()
          }
        }
        n118 = case shown="True" "INITIAL" {
          frame False {
          }
          frame True {
            n119 = call "Build Text9"("pwm3"="1500", "time"="1000", "pwm0"="1500", "pwm1"="1700", "pwm2"="1500", "pwm4"="1500") -> ("Result"=w210:string)  [unwired: 8 in, 1 out]
            n120 = local write "buffer"(w210) -> ()
            n121 = local write "PWM\nGRIPPER"(1600 ("Numeric")) -> ()
          }
        }
        n122 = call "Vision Acquisition"("Stop (F)"=w83) -> ("Image Out"=w95:T4, "Stopped"=w168:bool, "error out"=w165:errorcluster)  [unwired: 24 in]
        n123 = Unbundle By Name("Arm Dimensiions") -> ("l1"=w155:sgl, "l2"=w156:sgl, "l3"=w157:sgl, "l4"=w158:sgl)
        n124 = call-poly "VISA Configure Serial Port"("VISA resource name"="VISA NAME", "timeout (10sec)"=w143, "baud rate (9600)"=u32 115200 ("baud rate"), "data bits (8)"=u16 8 ("data bits"), "parity (0:none)"=w144, "stop bits (10: 1 bit)"=w142, "flow control (0:none)"=w141) -> ("VISA resource name out"=w139:refnum<visa-resource-name>, "error out"=w138:errorcluster)  [unwired: 7 in]
        n125 = case shown="True" TRUE ("WRITE") {
          tunnel: w139 -> [w525 w530]
          tunnel: w138 -> [w524 w529]
          tunnel: [w525 w528] -> w76
          tunnel: [w524 w527] -> w75
          tunnel: "buffer" -> [_ w526]
          frame False {
          }
          frame True {
            n126 = VISA Write(VISA resource name=w530, write buffer=w526, error in (no error)=w529) -> (VISA resource name out=w528:refnum<visa-resource-name>, error out=w527:errorcluster)  [unwired: 1 out]
          }
        }
        n127 = call "IMAQ ExtractSingleColorPlane"("Color Plane"=w166, "error in (no error)"=w165, "Image Dst"=w167, "Image Src"=w95) -> ("Image Dst Out"=w164:T4)  [unwired: 6 in, 1 out]
        n128 = call "Vision Assistant"("Image In"=w164, "error in"=w165) -> ("Edge Coordinates (horizontal)"=w110:cluster{"X":sgl, "Y":sgl}[], "Edge Coordinates (vertical)"=w109:cluster{"X":sgl, "Y":sgl}[], "error out"=w90:errorcluster)  [unwired: 20 in, 3 out]
        n129 = Array To Cluster(array=w110) -> (cluster=w111:T16)
        n130 = Array To Cluster(array=w109) -> (cluster=w108:T17)
        n131 = case shown="True" TRUE ("READ") {
          tunnel: w75 -> [w170 w187]
          tunnel: [w170 w182] -> w74
          tunnel: [w169 w183] -> w73
          tunnel: w76 -> [w169 w188]
          frame False {
          }
          frame True {
            # "Read the number of bytes specified."
            # "Write bytes to port."
            n132 = VISA Write(VISA resource name=w188, write buffer="va vb\n\r" ("string to write"), error in (no error)=w187) -> (VISA resource name out=w190:refnum<visa-resource-name>, error out=w192:errorcluster)  [unwired: 1 out]
            n133 = stacked-sequence {
              tunnel: w192 -> [w195]
              tunnel: [w195] -> w191
              tunnel: w190 -> [w194]
              tunnel: [w194] -> w189
              frame #0 {
                n134 = Wait (ms)(milliseconds to wait=u32 15 ("delay before read (ms)")) -> ()  [unwired: 1 out]
              }
            }
            n135 = property class="Instr"(reference=w189, error in=w191) -> (reference out=w180:refnum<visa-resource-name>, error out=w179:errorcluster, "Serial Settings:Number of Bytes at Serial Port"=w178:u32)
            "bytes read" <- w178
            n136 = VISA Read(VISA resource name=w180, byte count=w178, error in (no error)=w179) -> (VISA resource name out=w183:refnum<visa-resource-name>, read buffer=w185:string, error out=w182:errorcluster)  [unwired: 1 out]
            "read string" <- w185
            n137 = String To Byte Array(string=w185) -> (unsigned byte array=w186:u8[])
            n138 = Array To Cluster(array=w186) -> (cluster=w184:T18)
            n139 = Unbundle By Name(w184) -> ("unsigned byte array[0]"=w172:u8, "unsigned byte array[1]"=w171:u8)
            n140 = Greater Or Equal?(x=w172, y=w171) -> (x >= y?=w176:bool)
            n141 = Select(t=w172, s=w176, f=w171) -> (s? t:f=w175:u8)
            "INPUT" <- w175
            n142 = Greater Or Equal?(x=w175, y="SETPOINT\nGAYA") -> (x >= y?=w173:bool)
            n143 = local write "INDICATOR"(w173) -> ()
            n144 = Merge Signals(w172, w171, "SETPOINT\nGAYA") -> (→"Waveform Chart":dynamicdata)
          }
        }
        n145 = Unbundle By Name(w111) -> ("Edge Coordinates (horizontal)[0].X"=w67:sgl, "Edge Coordinates (horizontal)[1].X"=w71:sgl)
        n146 = Unbundle By Name(w108) -> ("Edge Coordinates (vertical)[0].Y"=w84:sgl, "Edge Coordinates (vertical)[1].Y"=w105:sgl)
        n147 = feedback #2() -> (w101:sgl)  [unwired: 1 in]
        n148 = Divide(x=w101, y=sgl 3.0) -> (x/y=w152:sgl)
        n149 = Subtract(x=w152, y=sgl 106.66667) -> (x-y=w131:sgl)
        "Y ROBOT" <- w131
        n150 = Greater Or Equal?(x=w84, y=sgl 120.0) -> (x >= y?=w107:bool)
        n151 = feedback #3() -> (w99:sgl)  [unwired: 1 in]
        n152 = Divide(x=w99, y=sgl 3.0) -> (x/y=w150:sgl)
        n153 = Add(x=w150, y=sgl 138.0) -> (x+y=w132:sgl)
        "X ROBOT" <- w132
        n154 = mathscript code="xr=abs(sqrt((X^2)+(Y^2)));\nx2=sin(deg_to_rad(offset))*l4;\nx1=xr-x2;\nz2=cos(deg_to_rad(offset))*l4;\nz1=z2+Z-l1;\nalpha=rad_to_deg(atan(z1/x1));\na=atan(z1/x1);\nTheta1=rad_to_deg(atan(Y/X));\nTheta2=rad_to_deg(abs((acos(((l3^2)-(l2^2)-(x1^2)-(z1^2))/(-2*l2*(sqrt((x1^2)+(z1^2)))))+a)));\nTheta3=rad_to_deg(abs((acos(((x1^2)+(z1^2)-(l3^2)-(l2^2))/(-2*l2*l3)))));\nTheta4=(270+offset)-alpha-(Theta2-alpha)-Theta3;\n\nj1x=0; j2x=0; j3x=cos(deg_to_rad(Theta2))*l2; j4x=x1; j5x=j4x+x2;\nj1z=0; j2z=l1; j3z=(sin(deg_to_rad(Theta2))*l2)+j2z; j4z=l1+z1; j5z=j4z-z2;\n\njt2x=0; jt3x=cos(deg_to_rad(Theta1))*j3x; jt4x=cos(deg_to_rad(Theta1))*j4x; jt5x=cos(deg_to_rad(Theta1))*j5x;\njt2y=0; jt3y=sin(deg_to_rad(Theta1))*j3x; jt4y=sin(deg_to_rad(Theta1))*j4x; jt5y=sin(deg_to_rad(Theta1))*j5x;;\n\nPW1=(-10*Theta1)+1500\nPW2=(9.555555556*Theta2)+630\nPW3=(-9.666666667*Theta3)+2640\nPW4=(10*Theta4)-400"("??"="error in", "X"=w132, "Y"=w131, "Z"=sgl 50.0, "l2"=w156, "l3"=w157, "l4"=w158, "l1"=w155, "offset"="OFFSET") -> ("??"=→"error out":errorcluster, "Theta1"=w61:dbl, "Theta2"=w60:dbl, "Theta3"=w59:dbl, "PW1"=w161:dbl, "PW2"=w160:dbl, "PW3"=w133:dbl, "j1x"=w57:i32, "j2x"=w56:i32, "j3x"=w55:dbl, "j4x"=w54:dbl, "j1z"=w52:i32, "j2z"=w51:sgl, "j3z"=w50:dbl, "j4z"=w49:dbl, "jt2x"=w47:i32, "jt3x"=w46:dbl, "jt4x"=w45:dbl, "jt2y"=w43:i32, "jt3y"=w42:dbl, "jt4y"=w41:dbl, "PW4"=w62:dbl, "Theta4"=w58:dbl, "j5x"=w53:dbl, "j5z"=w48:dbl, "jt5x"=w44:dbl, "jt5y"=w40:dbl)
        n155 = case shown="False" w107 {
          tunnel: w105 -> [_ w215]
          tunnel: w84 -> [w211 _]
          tunnel: [w212 w214] -> w87
          frame False {
            n156 = Subtract(x=w211, y=sgl 60.0) -> (x-y=w212:sgl)
          }
          frame True {
            n157 = Add(x=w215, y=sgl 60.0) -> (x+y=w214:sgl)
          }
        }
        n158 = Greater?(x=w87, y=sgl 0.0) -> (0:w126:bool)
        n159 = Greater?(x=w87, y=sgl 120.0) -> (0:w121:bool)
        n160 = Greater?(x=w87, y=sgl 340.0) -> (0:w116:bool)
        n161 = Less Or Equal?(x=w87, y=sgl 120.0) -> (x <= y?=w127:bool)
        n162 = Less Or Equal?(x=w87, y=sgl 340.0) -> (x <= y?=w122:bool)
        n163 = Less Or Equal?(x=w87, y=sgl 480.0) -> (x <= y?=w117:bool)
        n164 = And(x=w126, y=w127) -> (x .and. y?=w125:bool)
        n165 = And(x=w121, y=w122) -> (x .and. y?=w120:bool)
        n166 = And(x=w116, y=w117) -> (x .and. y?=w115:bool)
        n167 = case shown="True" w125 {
          frame False {
          }
          frame True {
            n168 = local write "OFFSET"(15.0 ("offset")) -> ()
          }
        }
        n169 = case shown="True" w120 {
          frame False {
          }
          frame True {
            n170 = local write "OFFSET"(60.0 ("offset")) -> ()
          }
        }
        n171 = case shown="True" w115 {
          frame False {
          }
          frame True {
            n172 = local write "OFFSET"(75.0 ("offset")) -> ()
          }
        }
        n173 = Greater?(x=w87, y=sgl 0.0) -> (0:w134:bool)
        n174 = Greater Or Equal?(x=w71, y=sgl 600.0) -> (x >= y?=w103:bool)
        n175 = case shown="True" w103 {
          tunnel: [w198 w202] -> w68
          tunnel: w71 -> [w197 _]
          tunnel: w67 -> [_ w200]
          frame False {
            n176 = Subtract(x=w197, y=sgl 60.0) -> (x-y=w198:sgl)
          }
          frame True {
            n177 = Add(x=w200, y=sgl 80.0) -> (x+y=w202:sgl)
          }
        }
        n178 = Greater?(x=w68, y=sgl 0.0) -> (0:w135:bool)
        n179 = And(x=w135, y=w134) -> (x .and. y?=w97:bool)
        n180 = case shown="False" w97 {
          tunnel: w68 -> [_ w533]
          tunnel: [w531 w534] -> w100
          tunnel: [w532 w533] -> w102
          tunnel: w87 -> [_ w534]
          tunnel: w101 -> [w532 _]
          tunnel: w99 -> [w531 _]
          frame False {
          }
          frame True {
          }
        }
        n181 = feedback-in #2(w102) -> ()
        n182 = feedback-in #3(w100) -> ()
        n183 = local read "START"() -> (w96:bool)
        n184 = Divide(x=w87, y=sgl 3.0) -> (x/y=→"Y CAMERA":sgl)
        n185 = Subtract(x=w68, y=w67) -> (x-y=w66:sgl)
        "SHADOW" <- w66
        n186 = Divide(x=w68, y=sgl 3.0) -> (x/y=→"X CAMERA":sgl)
        n187 = Build Array(w67, w84, w71, w105) -> (w112:sgl[])
        n188 = case shown="False" w96 {
          tunnel: w161 -> [w992 _]
          tunnel: w160 -> [w991 _]
          tunnel: w133 -> [w990 _]
          tunnel: w57 -> [w1018 _]
          tunnel: w56 -> [w1017 _]
          tunnel: w55 -> [w1016 _]
          tunnel: w54 -> [w1015 _]
          tunnel: w53 -> [w1014 _]
          tunnel: w52 -> [w1013 _]
          tunnel: w51 -> [w1012 _]
          tunnel: w50 -> [w1011 _]
          tunnel: w49 -> [w1010 _]
          tunnel: w48 -> [w1009 _]
          tunnel: w47 -> [w1005 _]
          tunnel: w46 -> [w1004 _]
          tunnel: w45 -> [w1003 _]
          tunnel: w44 -> [w1002 _]
          tunnel: w43 -> [w1001 _]
          tunnel: w42 -> [w1000 _]
          tunnel: w41 -> [w999 _]
          tunnel: w40 -> [w998 _]
          tunnel: w62 -> [w993 _]
          tunnel: w61 -> [w983 _]
          tunnel: w60 -> [w982 _]
          tunnel: w59 -> [w981 _]
          tunnel: w58 -> [w980 _]
          frame False {
            n189 = Build Array(w1005, w1004, w1003, w1002) -> (w1007:dbl[])
            n190 = Build Array(w1001, w1000, w999, w998) -> (w1006:dbl[])
            n191 = To Unsigned Long Integer(number=w992) -> (unsigned 32bit integer=w989:u32)
            n192 = To Unsigned Long Integer(number=w991) -> (unsigned 32bit integer=w987:u32)
            n193 = Build Array(w1018, w1017, w1016, w1015, w1014) -> (w1022:dbl[])
            n194 = To Unsigned Long Integer(number=w990) -> (unsigned 32bit integer=w986:u32)
            n195 = Build Array(w1013, w1012, w1011, w1010, w1009) -> (w1020:dbl[])
            n196 = To Unsigned Long Integer(number=w993) -> (unsigned 32bit integer=w985:u32)
            n197 = call "Convert to Dynamic Data3"("Array"=w1007) -> ("Dynamic Data Type"=w996:dynamicdata)  [unwired: 3 in]
            n198 = call "Convert to Dynamic Data4"("Array"=w1006) -> ("Dynamic Data Type"=w997:dynamicdata)  [unwired: 3 in]
            n199 = call "Convert to Dynamic Data"("Array"=w1022) -> ("Dynamic Data Type"=w1021:dynamicdata)  [unwired: 3 in]
            n200 = call "Convert to Dynamic Data2"("Array"=w1020) -> ("Dynamic Data Type"=w1019:dynamicdata)  [unwired: 3 in]
            n201 = Bundle By Name(cluster=T13 {"Theta1"=0.0, "Theta2"=0.0, "Theta3"=0.0, "Theta4"=0.0} ("Joint Angles"), "Theta1"=w983, "Theta2"=w982, "Theta3"=w981, "Theta4"=w980) -> (→"Joint Angles":T13)
            n202 = Bundle By Name(cluster=T12 {"PW1"=0, "PW2"=0, "PW3"=0, "PW4"=0} ("PWM Values 2"), "PW1"=w989, "PW2"=w987, "PW3"=w986, "PW4"=w985) -> (→"PWM Values":T12)
            n203 = call "Build XY Graph"("Y Input"=w1019, "X Input"=w1021) -> ("XY Graph"=→"SIDE VIEW":cluster{"Y":dbl[], "Y":dbl[]}[])  [unwired: 3 in, 6 out]
            n204 = call "Build XY Graph2"("Y Input"=w996, "X Input"=w997) -> ("XY Graph"=→"TOP VIEW":cluster{"Y":dbl[], "Y":dbl[]}[])  [unwired: 3 in, 6 out]
          }
          frame True {
          }
        }
        n205 = Array To Cluster(array=w112) -> (cluster=w94:T19)
        n206 = case shown="True" "FREEZE" {
          frame False {
          }
          frame True {
            n207 = local write "START"(FALSE ("START")) -> ()
          }
        }
        n208 = Subtract(x=sgl 720.0 ("Z CAMERA"), y=w67) -> (x-y=w70:sgl)
        n209 = call "IMAQ Overlay Rectangle"("Color"="Color", "error in (no error)"=w90, "Drawing Mode (Frame)"="Drawing Mode", "Rectangle"=w94, "Image"=w95) -> ("error out"=→"error vision":errorcluster, "Image Out"=→"Image":T4)  [unwired: 5 in]
        n210 = Multiply(x=sgl 480.0 ("Z CAMERA"), y=w66) -> (x*y=w79:sgl)
        n211 = Divide(x=w79, y=w70) -> (x/y=w77:sgl)
        n212 = VISA Close(VISA resource name=w73, error in (no error)=w74) -> (error out=w145:errorcluster)
        n213 = Divide(x=w77, y=sgl 3.0) -> (x/y=w64:sgl)
        "Z CAMERA" <- w64
        n214 = Divide(x=w64, y=sgl 1.0) -> (x/y=→"Z ROBOT":sgl)
        n215 = call <vilib>:"Simple Error Handler.vi"("error in (no error)"=w145) -> ()  [unwired: 4 in, 5 out]
      }
      frame False {
      }
    }
    n216 = Unbundle By Name("Dimensi Lengan Robot") -> ("l1"=w21:sgl, "l2"=w20:sgl, "l3"=w19:sgl, "l4"=w18:sgl)
    n217 = case shown="\"Kinematika Balik\"" "Kinematik Maju / Balik" {
      tunnel: [w1060 w1404] -> w26
      tunnel: [w1059 w1403] -> w25
      tunnel: [w1058 w1402] -> w24
      tunnel: [w1057 w1401] -> w23
      tunnel: w21 -> [w1056 w1400]
      tunnel: w20 -> [w1055 w1399]
      tunnel: w19 -> [w1054 w1398]
      tunnel: w18 -> [w1053 w1397]
      frame "Kinematika Maju", Default {
        n218 = mathscript code="Theta1=-q1;\nTheta2=q2;\nTheta3=q3;\nTheta4=q4;\n\nj1x=0; j2x=0; j3x=cos(deg_to_rad(Theta2))*l2; j4x=j3x+cos(deg_to_rad(270-(90-Theta2)+Theta3))*l3; j5x=j4x+cos(deg_to_rad(90-(90-Theta2-Theta3)+Theta4))*l4;\nj1z=0; j2z=l1; j3z=j2z+sin(deg_to_rad(Theta2))*l2; j4z=j3z+sin(deg_to_rad(270-(90-Theta2)+Theta3))*l3; j5z=j4z+sin(deg_to_rad(90-(90-Theta2-Theta3)+Theta4))*l4;\n\njt2x=0; jt3x=cos(deg_to_rad(Theta1))*j3x; jt4x=cos(deg_to_rad(Theta1))*j4x; jt5x=cos(deg_to_rad(Theta1))*j5x;\njt2y=0; jt3y=sin(deg_to_rad(Theta1))*j3x; jt4y=sin(deg_to_rad(Theta1))*j4x; jt5y=sin(deg_to_rad(Theta1))*j5x;\n\noffset=90+rad_to_deg((atan((j5z-j4z)/(j5x-j4x))));\n\nX=jt5x;\nY=-jt5y;\nZ=j5z;;"("q1"="BASE", "q2"="SHOULDER", "q3"="ELBOW", "l2"=w1055, "l3"=w1054, "l4"=w1053, "l1"=w1056, "q4"="WRIST") -> ("j1x"=w1042:i32, "j2x"=w1041:i32, "j3x"=w1040:dbl, "j4x"=w1039:dbl, "j1z"=w1037:i32, "j2z"=w1036:sgl, "j3z"=w1035:dbl, "j4z"=w1034:dbl, "jt2x"=w1032:i32, "jt3x"=w1031:dbl, "jt4x"=w1030:dbl, "jt2y"=w1028:i32, "jt3y"=w1027:dbl, "jt4y"=w1026:dbl, "X"=w1052:dbl, "Y"=w1051:dbl, "Z"=w1050:dbl, "offset"=w1043:dbl, "j5x"=w1038:dbl, "j5z"=w1033:dbl, "jt5x"=w1029:dbl, "jt5y"=w1025:dbl)  [unwired: 1 in, 1 out]
        n219 = Build Array(w1042, w1041, w1040, w1039, w1038) -> (w1060:dbl[])
        n220 = Build Array(w1037, w1036, w1035, w1034, w1033) -> (w1059:dbl[])
        n221 = Build Array(w1032, w1031, w1030, w1029) -> (w1058:dbl[])
        n222 = Build Array(w1028, w1027, w1026, w1025) -> (w1057:dbl[])
        n223 = Bundle(cluster=T14 {"Theta0"=0.0, "Theta1"=0.0, "Theta2"=0.0} ("Joint Angles"), "Theta0"=w1052, "Theta1"=w1051, "Theta2"=w1050) -> (→"Koordinat Akhir (KM)":T14)
        n224 = local write "theta"(w1043) -> ()
      }
      frame "Kinematika Balik" {
        # "Theta3 = atan2(D/-(sqrt(1-D^2))); \nTheta2=atan2(x1,z1)-atan2((l2+cos(deg_to_rad(Theta3))*l3),(sin(deg_to_rad(Theta3))*l3));"
        # "Enter constants for your servo calibrations here"
        n225 = Multiply(x="Koordinat Y", y=-1.0) -> (x*y=w1392:dbl)
        n226 = Select(t=1.0, s="ELBOW CONFIG", f=-1.0) -> (s? t:f=w1363:dbl)
        n227 = mathscript code="xr=abs(sqrt((X^2)+(Y^2)));\nx2=sin(deg_to_rad(offset))*l4;\nx1=xr-x2;\nz2=cos(deg_to_rad(offset))*l4;\nz1=z2+Z-l1;\nalpha=rad_to_deg(atan(z1/x1));\na=atan(z1/x1);\nTheta1=rad_to_deg(atan(Y/X));\nTheta2=rad_to_deg(a+notasi*acos(((l3^2)-(l2^2)-(x1^2)-(z1^2))/(-2*l2*(sqrt((x1^2)+(z1^2))))));\nTheta3=rad_to_deg(((acos(((x1^2)+(z1^2)-(l3^2)-(l2^2))/(-2*l2*l3)))));\nTheta4=(270+offset)-alpha-(Theta2-alpha)-Theta3;\n\nj1x=0; j2x=0; j3x=cos(deg_to_rad(Theta2))*l2; j4x=x1; j5x=j4x+x2;\nj1z=0; j2z=l1; j3z=(sin(deg_to_rad(Theta2))*l2)+j2z; j4z=l1+z1; j5z=j4z-z2;\n\njt2x=0; jt3x=cos(deg_to_rad(Theta1))*j3x; jt4x=cos(deg_to_rad(Theta1))*j4x; jt5x=cos(deg_to_rad(Theta1))*j5x;\njt2y=0; jt3y=sin(deg_to_rad(Theta1))*j3x; jt4y=sin(deg_to_rad(Theta1))*j4x; jt5y=sin(deg_to_rad(Theta1))*j5x;;"("X"="Koordinat X", "Y"=w1392, "Z"="Koordinat Z", "l2"=w1399, "l3"=w1398, "l4"=w1397, "l1"=w1400, "offset"="theta", "notasi"=w1363) -> ("Theta1"=w1390:dbl, "Theta2"=w1389:dbl, "Theta3"=w1388:dbl, "j1x"=w1384:i32, "j2x"=w1383:i32, "j3x"=w1382:dbl, "j4x"=w1381:dbl, "j1z"=w1379:i32, "j2z"=w1378:sgl, "j3z"=w1377:dbl, "j4z"=w1376:dbl, "jt2x"=w1374:i32, "jt3x"=w1373:dbl, "jt4x"=w1372:dbl, "jt2y"=w1370:i32, "jt3y"=w1369:dbl, "jt4y"=w1368:dbl, "Theta4"=w1387:dbl, "j5x"=w1380:dbl, "j5z"=w1375:dbl, "jt5x"=w1371:dbl, "jt5y"=w1367:dbl)  [unwired: 1 in, 1 out]
        n228 = Build Array(w1384, w1383, w1382, w1381, w1380) -> (w1404:dbl[])
        n229 = Build Array(w1379, w1378, w1377, w1376, w1375) -> (w1403:dbl[])
        n230 = Build Array(w1374, w1373, w1372, w1371) -> (w1402:dbl[])
        n231 = Build Array(w1370, w1369, w1368, w1367) -> (w1401:dbl[])
        n232 = Bundle(cluster=T15 {"Theta0"=0.0, "Theta1"=0.0, "Theta2"=0.0, "Theta3"=0.0} ("Joint Angles"), "Theta0"=w1390, "Theta1"=w1389, "Theta2"=w1388, "Theta3"=w1387) -> (→"Sudut Persendian (KB)":T15)
      }
    }
    n233 = case shown="False" "BERKAS / KAMERA" {
      tunnel: [w1777 w1780] -> w36
      tunnel: [w1778 w1779] -> w12
      frame True {
        n234 = call "Vision Acquisition3"() -> ("Image Out"=w1777:T4, "error out"=w1778:errorcluster)  [unwired: 25 in, 1 out]
      }
      frame False {
        n235 = call "Vision Acquisition2"("Image Path"="Alamat Berkas") -> ("Image Out"=w1780:T4, "error out"=w1779:errorcluster)  [unwired: 24 in, 1 out]
      }
    }
    "Citra Asli" <- w36
    n236 = call "IMAQ ExtractSingleColorPlane"("Color Plane"="Color Plane", "error in (no error)"=w12, "Image Dst"=w10, "Image Src"=w36) -> ("Image Dst Out"=w5:T4)  [unwired: 6 in, 1 out]
    "Citra \nHitam/Putih" <- w5
    n237 = call "IMAQ Threshold"("Replace Value"="Replace Value", "Keep/Replace Value (Replace)"=TRUE, "error in (no error)"=w12, "Range"="Range", "Image Src"=w5) -> ("Image Dst Out"=w4:T4)  [unwired: 5 in, 1 out]
    "Hasil\nSegmentasi" <- w4
    n238 = call "IMAQ Count Objects 2"("Settings"="Settings", "error in (no error)"=w12, "Image"=w4) -> ("error out"=→"error vision 2":errorcluster, "Number of Objects"=→"Number of Objects":i32, "Image Out"=→"Hasil \nKlasifikasi":T4, "Objects"=→"Objects":T5)  [unwired: 4 in, 1 out]
    n239 = call "Convert to Dynamic Data7"("Array"=w24) -> ("Dynamic Data Type"=w27:dynamicdata)  [unwired: 3 in]
    n240 = call "Convert to Dynamic Data8"("Array"=w23) -> ("Dynamic Data Type"=w28:dynamicdata)  [unwired: 3 in]
    n241 = call "Convert to Dynamic Data5"("Array"=w26) -> ("Dynamic Data Type"=w31:dynamicdata)  [unwired: 3 in]
    n242 = call "Convert to Dynamic Data6"("Array"=w25) -> ("Dynamic Data Type"=w30:dynamicdata)  [unwired: 3 in]
    n243 = call "Build XY Graph3"("Y Input"=w30, "X Input"=w31) -> ("XY Graph"=→"SIDE VIEW ROBOT":cluster{"Y":dbl[], "Y":dbl[]}[])  [unwired: 3 in, 6 out]
    n244 = call "Build XY Graph4"("Y Input"=w27, "X Input"=w28) -> ("XY Graph"=→"TOP VIEW ROBOT":cluster{"Y":dbl[], "Y":dbl[]}[])  [unwired: 3 in, 6 out]
  }
